vi "Front Panel.vi"() -> ()   [LabVIEW 2016]
panel:
  in  "Ip an Modem Switch":bool
  in  "Station Phone # or IP":string
  in  "Download":bool
  in  "End Date & Time":timestamp
  in  "Start Date & Time":timestamp
  # "Data Download Tool"
  # "Modem"
  # "IP"
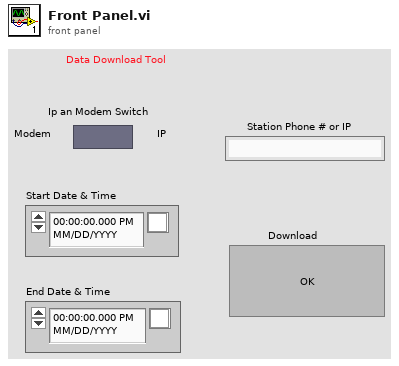
[diagram p1: front panel]
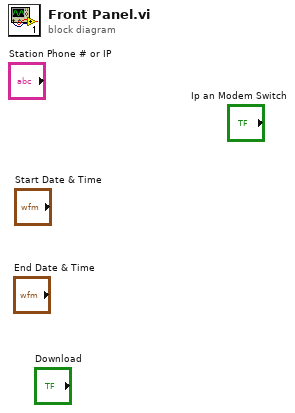
[diagram p0: block diagram]
diagram:
